vi "PE7260_Messgeraet.vi"(2 "refnum":refnum<file>) -> ()   [LabVIEW 2019]
uses:
  Global/Global Variables/Data_Display_global.vi
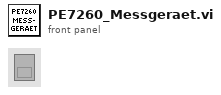
[diagram p1: front panel]
types:
  T1 = typedef "PE7265-Cluster.ctl" = cluster{"Lockin 1":dbl[][], "X1-Display":dbl, "X1 Percent":dbl, "Y1-Display":dbl, "X1 Percent 2":dbl, "Unit X1":string, "Unit X1a":string, "Unit X2":string, "Unit X2a":string, "X1 Overload":bool, "Y1 Overload":bool, "Sensitivity Setpoint":i16, "X1":dbl, "Y1":dbl}
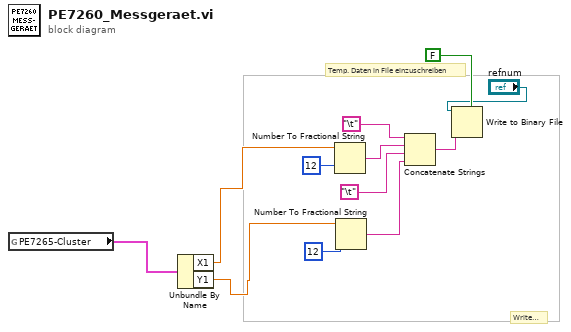
[diagram p0: block diagram]
diagram:
  # "Temp. Daten in File einzuschreiben"
  # "Write File"
  n1 = global read "Data_Display_global.vi" "PE7265-Cluster"() -> (w1:T1)
  n2 = Unbundle By Name(w1) -> ("X1"=w2:dbl, "Y1"=w3:dbl)
  n3 = Number To Fractional String(number=w2, precision (6)=i16 12) -> (F-format string=w10:string)  [unwired: 2 in]
  n4 = Number To Fractional String(number=w3, precision (6)=i16 12) -> (F-format string=w9:string)  [unwired: 2 in]
  n5 = Concatenate Strings("\t", w10, "\t", w9) -> (w12:string)
  n6 = Write to Binary File ("Write File")(file (use dialog)="refnum", data=w12, 5:FALSE ("prepend array or string size? (T)")) -> ()  [unwired: 3 in, 3 out]
